vi "SubVI_ChooseChannels.vi"(10 "String":string, 11 "Channel Selection":bool[](array[boolean])) -> (3 "Array":string[](array[string]))   [LabVIEW 2011]
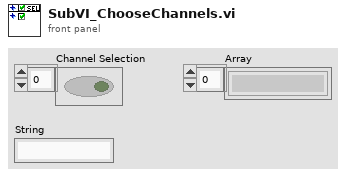
[diagram p1: front panel]
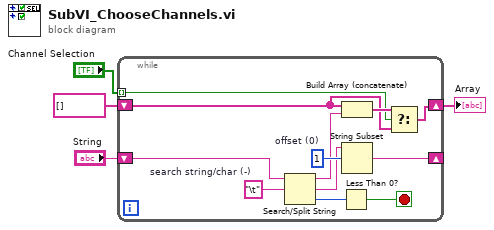
[diagram p0: block diagram]
diagram:
  n1 = while {
    shift-right: [w12] -> _
    shift-left: "String" -> [w16]
    tunnel: "Channel Selection" -> [w6] mode=indexing
    shift-right: [w7] -> w2
    shift-left: string[] [] -> [w5]
    stop <- w11 stop-if-true
    w14 = 1  # offset (0)
    w15 = "\t"  # search string/char (-)
    n2 = Search/Split String(string=w16, search string/char (-)=w15) -> (substring before match=w9:string, match + rest of string=w13:string, offset of match=w10:i32)  [unwired: 1 in]
    n3 = Less Than 0?(x=w10) -> (x < 0?=w11:bool)
    n4 = Build Array (concatenate)(w5, w9) -> (w8:string[])
    n5 = String Subset(string=w13, offset (0)=w14) -> (substring=w12:string)  [unwired: 1 in]
    n6 = Select(t=w8, s=w6, f=w5) -> (s? t:f=w7:string[])
  }
  "Array" <- w2
